vi "DefaultsGlobal.vi"() -> ()   [LabVIEW 2013, in "control module data interface generator.lvlib"]
uses:
  control module data interface generator.lvlib
panel:
  in  "Placeholder name":string="fmwk_placeholder"
  in  "Illegal Characters (regular expression)":string=">|<"
  # "edit this global to modify illegal characters and default placeholder names"
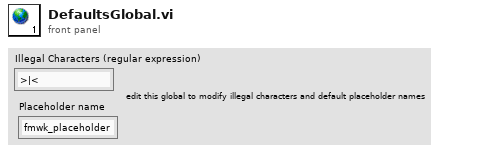
[diagram p1: front panel]
diagram:
